vi "Learn.vi"(9 "Learning?":bool=TRUE, 10 "cf":dbl, 11 "AER in":refnum<class "AER.lvclass">) -> (3 "AER out":refnum<class "AER.lvclass">)   [LabVIEW 2013, in "AER.lvclass"]
doc: "This VI implements the cerebellar learning algorithm"
uses:
  AER.lvclass
  AER.lvclass/AER.ctl
panel:
  out "WPFPC":dbl[](graph)
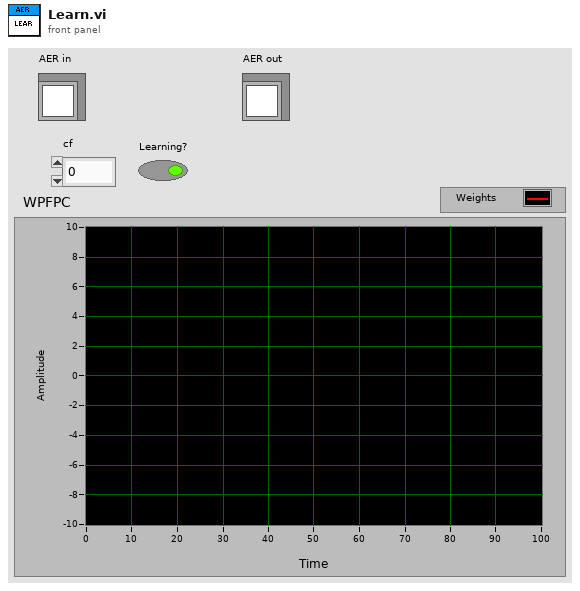
[diagram p1: front panel]
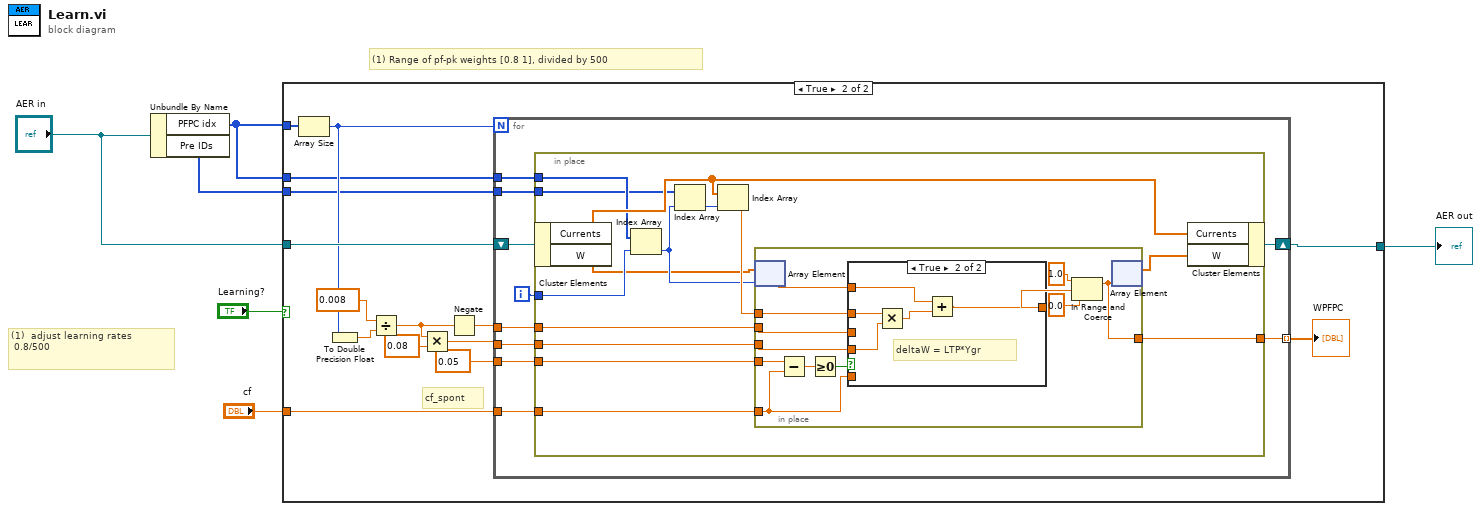
[diagram p0: block diagram]
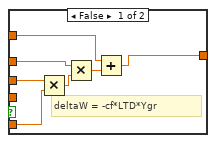
[diagram p3: hidden frame]
diagram:
  # "(1)  adjust learning rates\n 0.8/500"
  # "(1) Range of pf-pk weights [0.8 1], divided by 500"
  n1 = Unbundle By Name("AER in") -> ("PFPC idx"=w4:i32[], "Pre IDs"=w3:i32[])
  n2 = case shown="True" "Learning?" {
    tunnel: w4 -> [_ w22]
    tunnel: "AER in" -> [w7 w21]
    tunnel: [w7 w20] -> w1
    tunnel: "cf" -> [_ w19]
    tunnel: w4 -> [_ w11]
    tunnel: w3 -> [_ w10]
    frame False {
    }
    frame True {
      # "cf_spont"
      n3 = Array Size(array=w22) -> (size(s)=w14:i32)
      n4 = To Double Precision Float(number=w14) -> (double precision float=w9:dbl)
      n5 = Divide(x=0.008, y=w9) -> (x/y=w17:dbl)
      n6 = Multiply(x=w17, y=0.08) -> (x*y=w15:dbl)
      n7 = Negate(x=w17) -> (-x=w16:dbl)
      n8 = for {
        N: w14 -> [_]
        shift-right: [w32] -> w20
        shift-left: w21 -> [w28]
        tunnel: w19 -> [w31]
        tunnel: w15 -> [w30]
        tunnel: 0.05 ("x") -> [w29]
        tunnel: w16 -> [w26]
        tunnel: w11 -> [w25]
        tunnel: w10 -> [w24]
        tunnel: [w23] -> w8 mode=indexing
        i -> [w27]
        n9 = in-place {
          in-place-border: w31 -> [w46]
          in-place-border: w30 -> [w42]
          in-place-border: w29 -> [w45]
          in-place-border: w27 -> [w38]
          in-place-border: w26 -> [w41]
          in-place-border: w25 -> [w37]
          in-place-border: w24 -> [w36]
          in-place-border: [w33] -> w23
          n10 = in-place-cluster #1(w28) -> ("Currents"=w43:dbl[], "W"=w35:dbl[])
          n11 = Index Array(array=w37, index=w38) -> (element=w40:i32)
          n12 = Index Array(array=w36, index=w40) -> (element=w39:i32)
          n13 = Index Array(array=w43, index=w39) -> (element=w44:dbl)
          n14 = in-place {
            in-place-border: w46 -> [w52]
            in-place-border: w44 -> [w56]
            in-place-border: w45 -> [w58]
            in-place-border: w42 -> [w55]
            in-place-border: w41 -> [w54]
            in-place-border: [w47] -> w33
            n15 = in-place-array #2(w35, w40) -> (w51:dbl)
            n16 = Subtract(x=w58, y=w52) -> (x-y=w53:dbl)
            n17 = Greater Or Equal To 0?(x=w53) -> (x >= 0?=w57:bool)
            n18 = case shown="True" w57 {
              tunnel: w51 -> [w65 w70]
              tunnel: [w59 w66] -> w48
              tunnel: w56 -> [w64 w69]
              tunnel: w55 -> [_ w68]
              tunnel: w54 -> [w61 _]
              tunnel: w52 -> [w63 _]
              frame False {
                # "deltaW = -cf*LTD*Ygr"
                n19 = Multiply(x=w61, y=w63) -> (x*y=w62:dbl)
                n20 = Multiply(x=w64, y=w62) -> (x*y=w60:dbl)
                n21 = Add(x=w65, y=w60) -> (x+y=w59:dbl)
              }
              frame True {
                # "deltaW = LTP*Ygr"
                n22 = Multiply(x=w69, y=w68) -> (x*y=w67:dbl)
                n23 = Add(x=w70, y=w67) -> (x+y=w66:dbl)
              }
            }
            n24 = In Range and Coerce(upper limit=1.0, x=w48, lower limit=0.0) -> (coerced(x)=w47:dbl)  [unwired: 1 out]
            n25 = in-place-array #2(w47) -> (w34:dbl[])  [unwired: 1 out]
          }
          n26 = in-place-cluster #1("Currents"=w43, "W"=w34) -> (w32:refnum<class "AER.lvclass">)
        }
      }
      "WPFPC" <- w8
    }
  }
  "AER out" <- w1
